vi "Assert Greater Than or Equal To.vi"(5 "Expected":dbl, 7 "Message (\"\")":string, 8 "error in (no error)":errorcluster, 10 "Actual":dbl) -> (0 "error out":errorcluster)   [LabVIEW 2017, in "Transparent Assertions.lvlib"]
doc: "Asserts that a value is greater than or equal to the expected value. Returns an error if the assertion fails, and optionally appends a custom message to the error."
uses:
  Transparent Assertions.lvlib
  Logical Or/Logical Or.lvclass
  C:/Users/pasca/Projects/Home/TransparentAssertions/src/Transparent Assertions/Constraints/Binary Operator/Binary Operator.lvclass
  Is Greater Than/Is Greater Than.lvclass
  C:/Users/pasca/Projects/Home/TransparentAssertions/src/Transparent Assertions/Constraints/Constraint/Constraint.lvclass
  IsEqual/IsEqual.lvclass
  Binary Operator/Binary Operator.lvclass
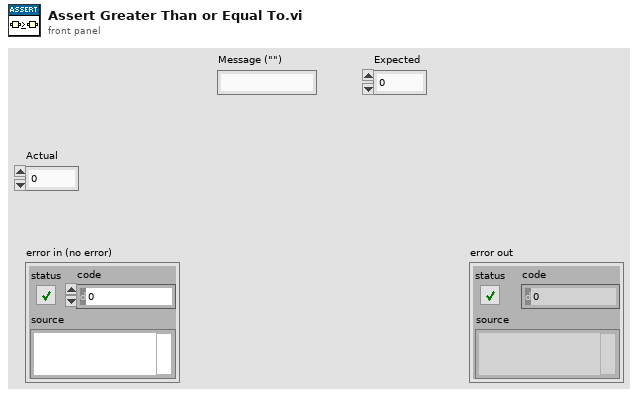
[diagram p1: front panel]
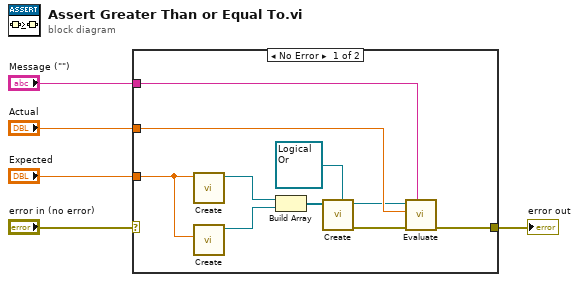
[diagram p0: block diagram]
diagram:
  n1 = case shown="No Error" "error in (no error)" {
    selector: "error in (no error)" -> [_ w16]
    tunnel: "Actual" -> [w15 _]
    tunnel: [w14 w16] -> w5
    tunnel: "Message (\"\")" -> [w13 _]
    tunnel: "Expected" -> [w12 _]
    frame No Error {
      n2 = call "Create.vi"("Expected"=w12) -> ("Is Greater Than"=w7:refnum<class "Is Greater Than.lvclass">)  [unwired: 9 in, 1 out]
      n3 = call "Create.vi"("Expected"=w12) -> ("IsEqual"=w8:refnum<class "IsEqual.lvclass">)  [unwired: 9 in, 1 out]
      n4 = Build Array(w7, w8) -> (w6:refnum<class "Constraint.lvclass">[])
      n5 = call "Create.vi"("Binary Operator in"=refnum<class "Logical Or.lvclass"> refnum ("Transparent Assertions.lvlib:Constraints.lvlib:Logical Or.lvclass"), "Constraints"=w6) -> ("error out"=w11:errorcluster, "Binary Operator"=w10:refnum<class "Logical Or.lvclass">)  [unwired: 8 in]
      n6 = call-dynamic "Evaluate.vi"("Message (\"\")"=w13, "error in (no error)"=w11, "Actual"=w15, "Constraint in"=w10) -> ("error out"=w14:errorcluster)  [unwired: 6 in, 1 out]
    }
    frame Error {
    }
  }
  "error out" <- w5
